vi "Start Step.vi"(8 "error in (no error)":errorcluster, 11 "Step in":refnum<class "Step.lvclass">) -> (0 "error out":errorcluster, 3 "Step out":refnum<class "Step.lvclass">)   [LabVIEW 2015, in "Step.lvclass"]
doc: "This VI is only run when starting a step"
uses:
  Step.lvclass
  Step.lvclass/Step.ctl
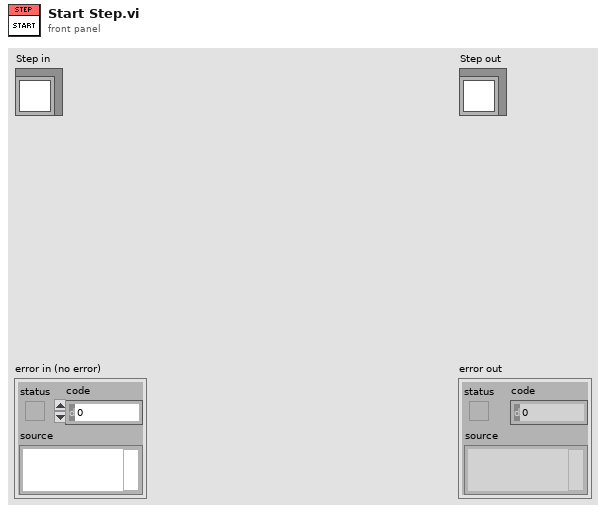
[diagram p1: front panel]
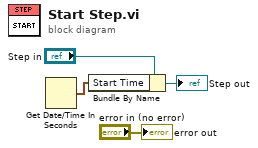
[diagram p0: block diagram]
diagram:
  n1 = Get Date/Time In Seconds() -> (seconds since 1Jan1904=w1:timestamp)
  n2 = Bundle By Name(cluster="Step in", "Start Time"=w1) -> (→"Step out":refnum<class "Step.lvclass">)
  "error out" <- "error in (no error)"
